vi "Change Y Axis.vi"(8 "error in (no error)":errorcluster, 11 "UI_Waveform in":refnum<class "UI_Waveform.lvclass">) -> (0 "error out":errorcluster, 3 "UI_Waveform out":refnum<class "UI_Waveform.lvclass">)   [LabVIEW 2021, in "UI_Waveform.lvclass"]
uses:
  UI_Waveform.lvclass
  UI_Waveform.lvclass/UI_Waveform.ctl
  <userlib>/_OpenG.lib/array/array.llb/Remove Duplicates from 1D Array (String)__ogtk.vi
panel:
  in  "Y Axie Name Array":string[](array[string])
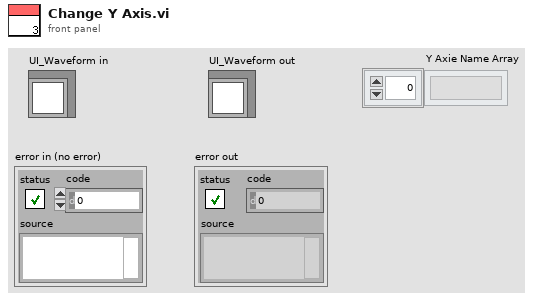
[diagram p1: front panel]
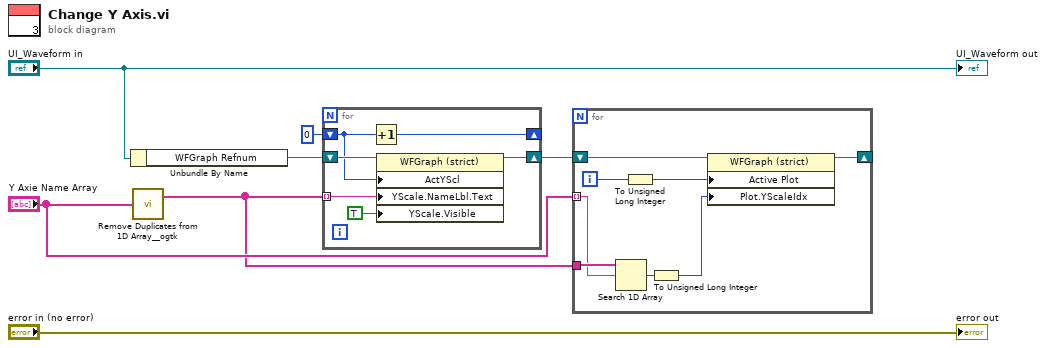
[diagram p0: block diagram]
diagram:
  n1 = Unbundle By Name("UI_Waveform in") -> ("WFGraph Refnum"=w4:refnum<vi>)
  n2 = call-poly <userlib>:"Remove Duplicates from 1D Array__ogtk.vi"("Input Array"="Y Axie Name Array") -> ("Output Array"=w1:string[])  [unwired: 1 out]
  n3 = for {
    shift-right: [w10] -> _
    shift-left: 0 ("Active Y Scale") -> [w11]
    tunnel: w1 -> [w9] mode=indexing
    shift-right: [w8] -> w3
    shift-left: w4 -> [w13]
    n4 = Increment(x=w11) -> (x+1=w10:i32)
    n5 = property class="WFGraph (strict)"(reference=w13, "ActYScl"=w11, "YScale.NameLbl.Text"=w9, "YScale.Visible"=TRUE ("Y Scale.Visible")) -> (reference out=w8:refnum<vi>)  [unwired: 1 in, 1 out]
  }
  n6 = for {
    tunnel: "Y Axie Name Array" -> [w16] mode=indexing
    shift-right: [w20] -> _
    shift-left: w3 -> [w21]
    tunnel: w1 -> [w17]
    i -> [w19]
    n7 = Search 1D Array(1D array=w17, element=w16) -> (index of element=w15:i32)  [unwired: 1 in]
    n8 = To Unsigned Long Integer(number=w19) -> (unsigned 32bit integer=w18:u32)
    n9 = To Unsigned Long Integer(number=w15) -> (unsigned 32bit integer=w14:u32)
    n10 = property class="WFGraph (strict)"(reference=w21, "Active Plot"=w18, "Plot.YScaleIdx"=w14) -> (reference out=w20:refnum<vi>)  [unwired: 1 in, 1 out]
  }
  "error out" <- "error in (no error)"
  "UI_Waveform out" <- "UI_Waveform in"
